vi "SearchAndCopy.vi"(8 "error in (no error)":errorcluster, 10 "SectionProperties":T1, 11 "ExistingFileMgr in":refnum<class "ExistingFileMgr.lvclass">) -> (0 "error out":errorcluster, 1 "Found index or EOF":bool, 2 "Existing File Chunk to copy":string, 3 "ExistingFileMgr out":refnum<class "ExistingFileMgr.lvclass">, 4 "Sweep Nums":i32[](array[numeric]), 5 "Next File Index":i64 format="%.9p", 6 "case":u32, 7 "starting File Index":i64 format="%.9p", 9 "Timestamps":i32[](array[numeric]))   [LabVIEW 2018, in "ExistingFileMgr.lvclass"]
doc: "Search for index in file where merge record belongs.\nCopy file prior to that index out to be saved in the new merge file."
uses:
  ExistingFileMgr.lvclass
  Sequence/SequenceSubvis/PolarizationSelect.ctl
  Sequence/SequenceSubvis/RF Direction.ctl
  Datalog/DatalogSubvis/SearchableTag.ctl
  Datalog/DataLog.lvclass
panel:
  out "error out 2":errorcluster
  out "Found Match or Insert index":bool
  # "1 match\n2 next record\n4 not found"
  # "debug"
  # "debug"
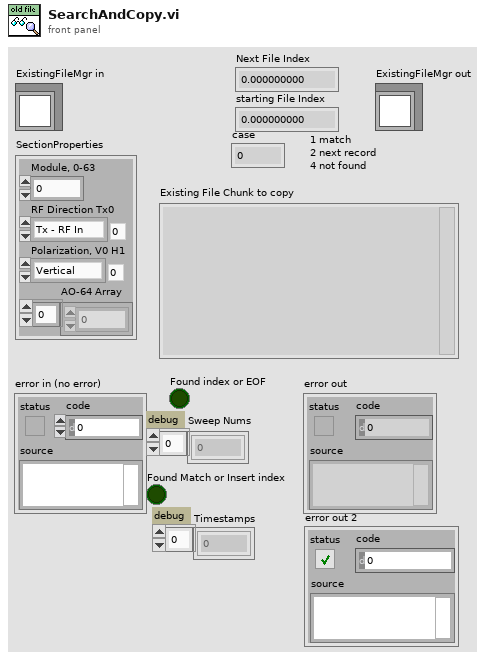
[diagram p1: front panel]
types:
  T1 = typedef "DataLog.lvclass/SearchableTag.ctl" = cluster{"Module, 0-63":i32, "RF Direction Tx0":T2, "Polarization, V0 H1":T3, "AO-64 Array":dbl[]}
  T2 = typedef "RF Direction.ctl" = enum16{"Tx - RF In", "Rx - RF Out"}
  T3 = typedef "PolarizationSelect.ctl" = enum16{"Vertical", "Horizontal"}
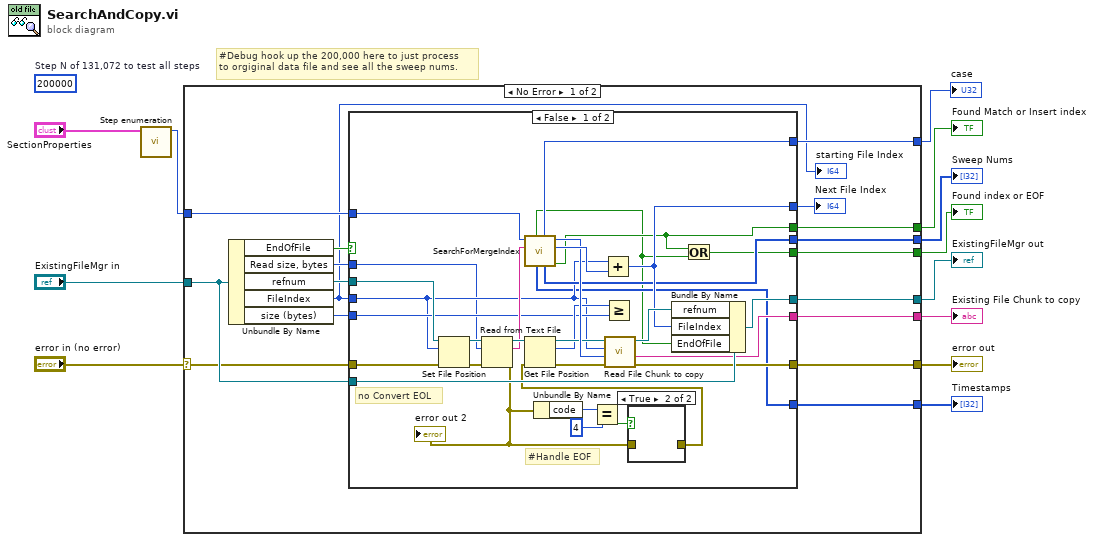
[diagram p0: block diagram]
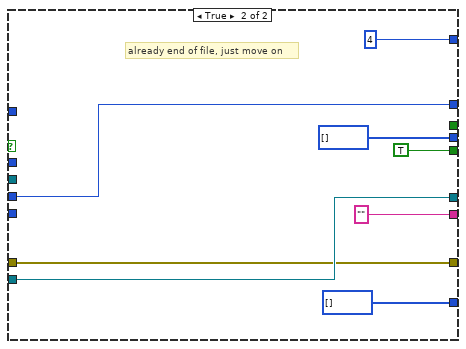
[diagram p3: hidden frame]
diagram:
  (unwired) 200000  # Step N of 131,072 to test all steps
  # "#Debug hook up the 200,000 here to just process\nto orgiginal data file and see all the sweep nums."
  n1 = call "Step enumeration.vi"("SweepProperties"="SectionProperties") -> ("Step N of 131,072"=w3:i32)  [unwired: 10 in]
  n2 = case shown="No Error" "error in (no error)" {
    selector: "error in (no error)" -> [w24 w72]
    tunnel: [w20 w72] -> w11
    tunnel: [w26 w71] -> w9
    tunnel: "ExistingFileMgr in" -> [w27 w71]
    tunnel: w3 -> [w28 _]
    tunnel: [w19 _] -> w7
    tunnel: [w18 _] -> w6
    tunnel: [w23 _] -> w5
    tunnel: [w21 _] -> w4
    tunnel: [w16 _] -> w2
    tunnel: [w13 _] -> w1
    frame No Error {
      n3 = Unbundle By Name(w27) -> ("EndOfFile"=w15:bool, "Read size, bytes"=w17:i32, "refnum"=w29:refnum<file>, "FileIndex"=w14:i64, "size (bytes)"=w22:i64)
      "starting File Index" <- w14
      n4 = case shown="False" w15 {
        tunnel: w29 -> [w61 _]
        tunnel: w28 -> [w60 _]
        tunnel: w27 -> [w59 w70]
        tunnel: [w58 w70] -> w26
        tunnel: [w52 w65] -> w25
        tunnel: w24 -> [w50 w69]
        tunnel: [w47 i32[] [] ("sweep record numbers")] -> w23
        tunnel: w22 -> [w45 _]
        tunnel: [w44 TRUE] -> w21
        tunnel: [w42 w69] -> w20
        tunnel: [w41 "" ("File body to copy")] -> w19
        tunnel: w14 -> [w35 w65]
        tunnel: [w34 _] -> w18
        tunnel: w17 -> [w33 _]
        tunnel: [w32 u32 4 ("case")] -> w16
        tunnel: [w31 i32[] [] ("sweep record numbers")] -> w13
        frame False {
          # "#Handle EOF"
          # "no Convert EOL"
          n5 = Set File Position(offset (in bytes) (0)=w35, refnum=w61, error in=w50) -> (refnum out=w55:refnum<file>, error out=w56:errorcluster)  [unwired: 1 in]
          n6 = Read from Text File(file (use dialog)=w55, count=w33, error in=w56) -> (refnum out=w54:refnum<file>, text=w49:string, error out=w36:errorcluster)  [unwired: 1 in, 1 out]
          "error out 2" <- w36
          n7 = call "SearchForMergeIndex.vi"("text"=w49, "Step N of 131,072"=w60) -> ("Found Match or Insert"=w34:bool, "incr file index"=w53:i64, "copy length"=w51:i32, "sweep record numbers"=w47:i32[], "case"=w32:u32, "Timestamps"=w31:i32[], "ENDOFFILE"=w30:bool)  [unwired: 2 in, 1 out]
          n8 = Unbundle By Name(w36) -> ("code"=w40:i32)
          n9 = Equal?(x=w40, y=4) -> (x = y?=w38:bool)
          n10 = Add(x=w35, y=w53) -> (x+y=w52:i64)
          n11 = case shown="True" w38 {
            tunnel: w36 -> [w62 _]
            tunnel: [w62 _] -> w37
            frame False {
            }
            frame True {
            }
          }
          n12 = Get File Position(4:w37, 7:w54) -> (0:w43:errorcluster, 2:w46:i64, 3:w48:refnum<file>)
          n13 = Greater Or Equal?(x=w46, y=w45) -> ()  [unwired: 1 out]
          n14 = call "Read File Chunk to copy.vi"("error in"=w43, "Length to copy"=w51, "Start index"=w35, "refnum"=w48) -> ("error out"=w42:errorcluster, "File body to copy"=w41:string, "refnum out"=w57:refnum<file>)  [unwired: 5 in]
          n15 = Bundle By Name(cluster=w59, "refnum"=w57, "FileIndex"=w52, "EndOfFile"=w30) -> (w58:refnum<class "ExistingFileMgr.lvclass">)
          n16 = Or(x=w34, y=w30) -> (x .or. y?=w44:bool)
        }
        frame True {
          # "already end of file, just move on"
        }
      }
      "Next File Index" <- w25
    }
    frame Error {
    }
  }
  "error out" <- w11
  "ExistingFileMgr out" <- w9
  "Existing File Chunk to copy" <- w7
  "Found Match or Insert index" <- w6
  "Sweep Nums" <- w5
  "Found index or EOF" <- w4
  "case" <- w2
  "Timestamps" <- w1
